vi "log analysis_gps.vi"() -> ()   [LabVIEW 2018] (continued)
15:20:57.4\tlog_raw\tgps_raw\t#DUALANTENNAHEADINGA,USB3,0,49.5,FINESTEERING,2107,282075.400,02000000,d426,15824;SOL_COMPUTED,L1_FLOAT,-1.000000000,190.728332520,52.272701263,0.0,209.958755493,180.000000000,\"631T\",21,7,7,7,04,00,20,02*2a740797\n\tsystem status\tnormal 2 28.100000 0 0\trobot status\t246.921443\t96.474986\t8.494500\t0.148213\t0.043685\t-28.674334\t0.301000\t0.002000\n\t\n15:20:57.9\tlog_raw\tgps_raw\t#DUALANTENNAHEADINGA,USB3,0,49.5,FINESTEERING,2107,282075.900,02000000,d426,15824;SOL_COMPUTED,L1_FLOAT,-1.000000000,190.868621826,51.534015656,0.0,206.683425903,180.000000000,\"631T\",14,7,7,7,04,00,20,03*060951e8\n\tsystem status\tnormal 2 28.100000 0 0\trobot status\t247.040258\t96.400033\t8.497000\t0.123898\t-0.129590\t-28.934715\t0.297000\t-0.013000\n\t\n15:20:58.4\tlog_raw\tgps_raw\t#DUALANTENNAHEADINGA,USB3,0,44.0,FINESTEERING,2107,282076.400,02000000,d426,15824;SOL_COMPUTED,NARROW_FLOAT,-1.000000000,164.765243530,-0.145935059,0.0,360.000000000,180.000000000,\"631T\",15,7,7,7,04,00,20,03*df327d6c\n\tsystem status\tnormal 2 28.100000 0 0\trobot status\t247.153173\t96.328172\t8.499300\t0.054880\t0.026721\t-29.154516\t0.311000\t0.002000\n\t\n15:20:58.9\tlog_raw\tgps_raw\t\tsystem status\tnormal 2 28.100000 0 0\trobot status\t247.265732\t96.255208\t8.500200\t0.112861\t0.355298\t-29.271130\t0.297000\t0.005000\n\t\n15:20:59.4\tlog_raw\tgps_raw\t\tsystem status\tnormal 2 28.100000 0 0\trobot status\t247.378509\t96.180954\t8.500400\t0.252561\t0.434005\t-29.420749\t0.301000\t0.008000\n\t\n15:20:59.9\tlog_raw\tgps_raw\t#DUALANTENNAHEADINGA,USB3,0,48.0,FINESTEERING,2107,282077.900,02000000,d426,15824;SOL_COMPUTED,NARROW_FLOAT,-1.000000000,163.219406128,-2.743896484,0.0,360.000000000,180.000000000,\"631T\",17,7,7,7,04,00,20,03*74221424\n\tsystem status\tnormal 2 28.100000 0 0\trobot status\t247.489808\t96.106361\t8.500700\t0.444252\t0.467575\t-29.545531\t0.301000\t0.005000\n\t\n15:21:00.4\tlog_raw\tgps_raw\t#DUALANTENNAHEADINGA,USB3,0,48.5,FINESTEERING,2107,282078.400,02000000,d426,15824;SOL_COMPUTED,NARROW_FLOAT,-1.000000000,164.756866455,-2.259979248,0.0,360.000000000,180.000000000,\"631T\",19,7,7,7,04,00,20,03*e2d4ab8a\n\tsystem status\tnormal 2 28.100000 0 0\trobot status\t247.603389\t96.030616\t8.501500\t0.397812\t0.362126\t-29.601914\t0.298000\t0.011000\n\t\n15:21:00.9\tlog_raw\tgps_raw\t#DUALANTENNAHEADINGA,USB3,0,48.5,FINESTEERING,2107,282078.900,02000000,d426,15824;SOL_COMPUTED,NARROW_FLOAT,-1.000000000,165.064834595,-2.246643066,0.0,360.000000000,180.000000000,\"631T\",18,7,7,7,04,00,20,03*e6e75529\n\tsystem status\tnormal 2 28.100000 0 0\trobot status\t247.723401\t95.952238\t8.502900\t0.211029\t0.110570\t-29.619450\t0.309000\t0.029000\n\t\n15:21:01.4\tlog_raw\tgps_raw\t#DUALANTENNAHEADINGA,USB3,0,47.5,FINESTEERING,2107,282079.400,02000000,d426,15824;SOL_COMPUTED,NARROW_FLOAT,-1.000000000,174.896926880,-30.356231689,0.0,360.000000000,180.000000000,\"631T\",18,7,7,7,04,00,20,03*d638673a\n\tsystem status\tnormal 2 28.100000 0 0\trobot status\t247.845096\t95.872152\t8.504300\t0.085021\t-0.119901\t-29.645623\t0.305000\t0.015000\n\t\n15:21:01.9\tlog_raw\tgps_raw\t#DUALANTENNAHEADINGA,USB3,0,47.5,FINESTEERING,2107,282079.900,02000000,d426,15824;SOL_COMPUTED,NARROW_FLOAT,-1.000000000,174.578781128,-31.075134277,0.0,360.000000000,180.000000000,\"631T\",17,7,7,7,04,00,20,03*d8acf742\n\tsystem status\tnormal 2 28.100000 0 0\trobot status\t247.963689\t95.793632\t8.505400\t-0.028469\t-0.053955\t-29.669528\t0.311000\t0.004000\n\t\n15:21:02.4\tlog_raw\tgps_raw\t\tsystem status\tnormal 2 28.100000 0 0\trobot status\t248.081422\t95.714785\t8.506300\t0.031084\t0.050569\t-29.647929\t0.294000\t0.017000\n\t\n15:21:02.9\tlog_raw\tgps_raw\t\tsystem status\tnormal 2 28.000000 0 0\trobot status\t248.195751\t95.637362\t8.506100\t0.171329\t0.096604\t-29.343964\t0.370000\t-0.086000\n\t\n15:21:03.4\tlog_raw\tgps_raw\t#DUALANTENNAHEADINGA,USB3,0,48.5,FINESTEERING,2107,282081.400,02000000,d426,15824;SOL_COMPUTED,NARROW_FLOAT,-1.000000000,186.002395630,72.538307190,0.0,360.000000000,180.000000000,\"631T\",18,7,7,7,04,00,20,02*94d40da5\n\tsystem status\tnormal 2 28.000000 0 0\trobot status\t248.312016\t95.561491\t8.506800\t0.012488\t0.198787\t-29.021105\t0.344000\t-0.051000\n\t\n15:21:03.9\tlog_raw\tgps_raw\t\tsystem status\tnormal 2 27.900000 0 0\trobot status\t248.431222\t95.484532\t8.507600\t-0.122842\t0.122402\t-28.483538\t0.262000\t0.063000\n\t\n15:21:04.4\tlog_raw\tgps_raw\t\tsystem status\tnormal 2 27.900000 0 0\trobot status\t248.548442\t95.409781\t8.509600\t-0.163692\t0.149809\t-27.878037\t0.300000\t0.006000\n\t\n15:21:04.9\tlog_raw\tgps_raw\t\tsystem status\tnormal 2 28.000000 0 0\trobot status\t248.667064\t95.335298\t8.510200\t-0.079262\t0.300498\t-27.192799\t0.222000\t0.147000\n\t\n15:21:05.4\tlog_raw\tgps_raw\t#INSPVAXA,USB3,0,48.0,FINESTEERING,2107,282083.450,02000000,471d,15824;INS_ALIGNMENT_COMPLETE,INS_RTKFIXED,37.37098848557,126.72364391635,8.5085,22.3000,-0.1545,0.2353,-0.0017,0.125081225,0.334802471,116.544491320,0.3966,0.2931,0.5085,0.1074,0.0919,0.0749,0.1481,0.1501,5.0097,0f000001,0*707b4fda\n\tsystem status\tnormal 2 28.000000 0 0\trobot status\t248.799900\t95.253167\t8.508500\t0.125081\t0.334802\t-26.544491\t0.294000\t0.032000\n\t\n15:21:05.9\tlog_raw\tgps_raw\t#INSPVAXA,USB3,0,48.0,FINESTEERING,2107,282083.950,02000000,471d,15824;INS_ALIGNMENT_COMPLETE,INS_RTKFIXED,37.37098781334,126.72364531945,8.5061,22.3000,-0.1397,0.2470,-0.0039,0.130744788,0.168821644,116.045699984,0.3966,0.2931,0.5085,0.1074,0.0919,0.0749,0.1481,0.1501,5.0097,0f000001,0*8c7cd4e3\n\tsystem status\tnormal 2 27.900000 0 0\trobot status\t248.924184\t95.178556\t8.506100\t0.130745\t0.168822\t-26.045700\t0.306000\t0.015000\n\t\n15:21:06.4\tlog_raw\tgps_raw\t#INSPVAXA,USB3,0,49.5,FINESTEERING,2107,282084.450,02000000,471d,15824;INS_ALIGNMENT_COMPLETE,INS_RTKFIXED,37.37098717814,126.72364671785,8.5044,22.3000,-0.1354,0.2435,-0.0138,-0.054756889,-0.022563669,115.524105800,0.3967,0.2930,0.5082,0.1073,0.0917,0.0749,0.1480,0.1501,5.0101,0f000001,0*e14fe85b\n\tsystem status\tnormal 2 28.000000 0 0\trobot status\t249.048052\t95.108055\t8.504400\t-0.054757\t-0.022564\t-25.524106\t0.397000\t-0.137000\n\t\n15:21:06.9\tlog_raw\tgps_raw\t#DUALANTENNAHEADINGA,USB3,0,49.5,FINESTEERING,2107,282084.900,02000000,d426,15824;SOL_COMPUTED,NARROW_FLOAT,-1.000000000,161.093994141,-39.642028809,0.0,360.000000000,180.000000000,\"631T\",18,7,7,7,04,00,20,02*551afc73\n\tsystem status\tnormal 2 28.000000 0 0\trobot status\t249.161436\t95.044023\t8.503800\t-0.170407\t-0.184756\t-25.155498\t0.339000\t-0.036000\n\t\n15:21:07.4\tlog_raw\tgps_raw\t\tsystem status\tnormal 2 28.000000 0 0\trobot status\t249.290152\t94.971247\t8.503100\t-0.112588\t-0.413886\t-24.896418\t0.198000\t0.158000\n\t\n15:21:07.9\tlog_raw\tgps_raw\t\tsystem status\tnormal 2 28.000000 0 0\trobot status\t249.416871\t94.899708\t8.501000\t-0.049468\t-0.480154\t-24.681244\t0.257000\t0.076000\n\t\n15:21:08.4\tlog_raw\tgps_raw\t\tsystem status\tnormal 2 28.000000 0 0\trobot status\t249.543697\t94.830890\t8.500800\t-0.123153\t-0.405635\t-24.666717\t0.251000\t0.079000\n\t\n15:21:08.9\tlog_raw\tgps_raw\t#INSPVAXA,USB3,0,45.5,FINESTEERING,2107,282086.950,02000000,471d,15824;INS_ALIGNMENT_COMPLETE,INS_RTKFIXED,37.37098400291,126.72365390857,8.5011,22.3000,-0.1413,0.2614,-0.0071,-0.222662760,-0.431667529,114.703885924,0.3961,0.2927,0.5077,0.1073,0.0916,0.0749,0.1479,0.1501,5.0112,0f000001,0*8c0cd5e8\n\tsystem status\tnormal 2 28.100000 0 0\trobot status\t249.684995\t94.755634\t8.501100\t-0.222663\t-0.431668\t-24.703886\t0.253000\t0.069000\n\t\n15:21:09.4\tlog_raw\tgps_raw\t\tsystem status\tnormal 2 28.100000 0 0\trobot status\t249.796178\t94.694217\t8.502700\t-0.161427\t-0.370643\t-24.781443\t0.302000\t-0.009000\n\t\n15:21:09.9\tlog_raw\tgps_raw\t#INSPVAXA,USB3,0,49.0,FINESTEERING,2107,282087.950,02000000,471d,15824;INS_ALIGNMENT_COMPLETE,INS_RTKFIXED,37.37098277282,126.72365670812,8.5043,22.3000,-0.1437,0.2560,-0.0135,-0.068385407,-0.323416769,114.901118705,0.3958,0.2926,0.5076,0.1072,0.0916,0.0749,0.1479,0.1502,5.0118,0f000001,0*c54dad40\n\tsystem status\tnormal 2 28.100000 0 0\trobot status\t249.932974\t94.619105\t8.504300\t-0.068385\t-0.323417\t-24.901119\t0.298000\t-0.013000\n\t\n15:21:10.4\tlog_raw\tgps_raw\t#INSPVAXA,USB3,0,45.0,FINESTEERING,2107,282088.450,02000000,471d,15824;INS_ALIGNMENT_COMPLETE,INS_RTKFIXED,37.37098213793,126.72365811830,8.5048,22.3000,-0.1404,0.2509,-0.0150,-0.140571199,-0.324537767,115.053900448,0.3958,0.2925,0.5075,0.1072,0.0917,0.0749,0.1479,0.1502,5.0126,0f000001,0*5d76f850\n\tsystem status\tnormal 2 28.100000 0 0\trobot status\t250.057886\t94.548639\t8.504800\t-0.140571\t-0.324538\t-25.053900\t0.300000\t-0.020000\n\t\n15:21:10.9\tlog_raw\tgps_raw\t\tsystem status\tnormal 2 28.100000 0 0\trobot status\t250.170070\t94.483065\t8.505900\t-0.049148\t-0.443713\t-25.152133\t0.309000\t-0.009000\n\t\n15:21:11.4\tlog_raw\tgps_raw\t\tsystem status\tnormal 2 28.100000 0 0\trobot status\t250.293447\t94.411259\t8.508800\t-0.003833\t-0.433412\t-25.288607\t0.296000\t-0.018000\n\t\n15:21:11.9\tlog_raw\tgps_raw\t#INSPVAXA,USB3,0,50.0,FINESTEERING,2107,282089.950,02000000,471d,15824;INS_ALIGNMENT_COMPLETE,INS_RTKFIXED,37.37098017514,126.72366234895,8.5129,22.3000,-0.1403,0.2638,-0.0115,0.068877400,-0.331025917,115.512688537,0.3958,0.2925,0.5074,0.1072,0.0917,0.0749,0.1479,0.1501,5.0134,0f000001,0*45d8cdd7\n\tsystem status\tnormal 2 28.100000 0 0\trobot status\t250.432630\t94.330788\t8.512900\t0.068877\t-0.331026\t-25.512689\t0.298000\t-0.016000\n\t\n15:21:12.4\tlog_raw\tgps_raw\t#INSPVAXA,USB3,0,47.0,FINESTEERING,2107,282090.450,02000000,471d,15824;INS_ALIGNMENT_COMPLETE,INS_RTKFIXED,37.37097950653,126.72366381280,8.5149,22.3000,-0.1497,0.2592,-0.0041,-0.040058431,-0.070783873,115.696569109,0.3958,0.2925,0.5072,0.1072,0.0918,0.0748,0.1480,0.1501,5.0142,0f000001,0*06fd62fb\n\tsystem status\tnormal 2 28.100000 0 0\trobot status\t250.562295\t94.256579\t8.514900\t-0.040058\t-0.070784\t-25.696569\t0.295000\t-0.015000\n\t\n15:21:12.9\tlog_raw\tgps_raw\t#DUALANTENNAHEADINGA,USB3,0,47.0,FINESTEERING,2107,282090.900,02000000,d426,15824;SOL_COMPUTED,NARROW_FLOAT,-1.000000000,171.721908569,34.681911469,0.0,360.000000000,180.000000000,\"631T\",20,7,7,7,04,00,20,03*da0d38e5\n\tsystem status\tnormal 2 28.100000 0 0\trobot status\t250.677266\t94.189308\t8.516000\t-0.049841\t0.271250\t-25.895908\t0.306000\t-0.016000\n\t\n15:21:13.4\tlog_raw\tgps_raw\t#INSPVAXA,USB3,0,47.0,FINESTEERING,2107,282091.450,02000000,471d,15824;INS_ALIGNMENT_COMPLETE,INS_RTKFIXED,37.37097820755,126.72366660545,8.5215,22.3000,-0.1497,0.2548,0.0005,-0.143132038,0.926627328,116.158649383,0.3959,0.2925,0.5072,0.1072,0.0918,0.0748,0.1480,0.1501,5.0152,0f000001,0*c99bd82f\n\tsystem status\tnormal 2 28.100000 0 0\trobot status\t250.809663\t94.112405\t8.521500\t-0.143132\t0.926627\t-26.158649\t0.299000\t-0.014000\n\t\n15:21:13.9\tlog_raw\tgps_raw\t#DUALANTENNAHEADINGA,USB3,0,47.0,FINESTEERING,2107,282091.900,02000000,d426,15824;SOL_COMPUTED,NARROW_FLOAT,-1.000000000,112.916130066,31.135679245,0.0,360.000000000,180.000000000,\"631T\",17,8,8,7,04,00,20,03*e78407cb\n\tsystem status\tnormal 2 28.100000 0 0\trobot status\t250.929101\t94.041496\t8.525700\t-0.018408\t0.996780\t-26.393163\t0.310000\t-0.006000\n\t\n15:21:14.4\tlog_raw\tgps_raw\t\tsystem status\tnormal 2 28.100000 0 0\trobot status\t251.054651\t93.967882\t8.529200\t-0.147378\t0.978647\t-26.703970\t0.302000\t-0.013000\n\t\n15:21:14.9\tlog_raw\tgps_raw\t#INSPVAXA,USB3,0,44.5,FINESTEERING,2107,282092.950,02000000,471d,15824;INS_ALIGNMENT_COMPLETE,INS_RTKFIXED,37.37097614467,126.72367094542,8.5349,22.3000,-0.1554,0.2816,0.0034,-0.093672408,0.920148848,117.196010792,0.3968,0.2926,0.5073,0.1073,0.0918,0.0749,0.1480,0.1500,5.0167,0f000001,0*78c5bf02\n\tsystem status\tnormal 2 28.100000 0 0\trobot status\t251.194091\t93.883445\t8.534900\t-0.093672\t0.920149\t-27.196011\t0.271000\t-0.056000\n\t\n15:21:15.4\tlog_raw\tgps_raw\t#INSPVAXA,USB3,0,49.0,FINESTEERING,2107,282093.450,02000000,471d,15824;INS_ALIGNMENT_COMPLETE,INS_RTKFIXED,37.37097543650,126.72367235664,8.5399,22.3000,-0.1638,0.2823,0.0033,-0.126887111,0.570236621,117.700862791,0.3975,0.2926,0.5072,0.1072,0.0917,0.0749,0.1480,0.1500,5.0184,0f000001,0*ead874db\n\tsystem status\tnormal 2 28.100000 0 0\trobot status\t251.319094\t93.804845\t8.539900\t-0.126887\t0.570237\t-27.700863\t0.283000\t-0.053000\n\t\n15:21:15.9\tlog_raw\tgps_raw\t#DUALANTENNAHEADINGA,USB3,0,49.0,FINESTEERING,2107,282093.900,02000000,d426,15824;SOL_COMPUTED,NARROW_FLOAT,-1.000000000,156.493606567,-47.281768799,0.0,360.000000000,180.000000000,\"631T\",19,7,7,7,04,00,20,03*77a80aac\n\tsystem status\tnormal 2 28.000000 0 0\trobot status\t251.432949\t93.733402\t8.545000\t-0.389248\t0.357754\t-28.088524\t0.278000\t-0.065000\n\t\n15:21:16.4\tlog_raw\tgps_raw\t\tsystem status\tnormal 2 28.000000 0 0\trobot status\t251.554090\t93.656544\t8.548800\t-0.417645\t0.623151\t-28.489175\t0.270000\t-0.059000\n\t\n15:21:16.9\tlog_raw\tgps_raw\t\tsystem status\tnormal 2 28.000000 0 0\trobot status\t251.675834\t93.577949\t8.555400\t-0.297721\t0.578023\t-28.861659\t0.303000\t-0.034000\n\t\n15:21:17.4\tlog_raw\tgps_raw\t\tsystem status\tnormal 2 28.100000 0 0\trobot status\t251.794007\t93.497874\t8.561500\t-0.057927\t0.756210\t-29.237305\t0.346000\t0.056000\n\t\n15:21:17.9\tlog_raw\tgps_raw\t\tsystem status\tnormal 2 28.100000 0 0\trobot status\t251.912469\t93.418342\t8.568300\t0.007452\t0.966597\t-29.571126\t0.263000\t-0.068000\n\t\n15:21:18.4\tlog_raw\tgps_raw\t\tsystem status\tnormal 2 28.100000 0 0\trobot status\t252.031352\t93.338903\t8.575100\t-0.062826\t1.099209\t-29.892121\t0.312000\t0.017000\n\t\n15:21:18.9\tlog_raw\tgps_raw\t#INSPVAXA,USB3,0,47.0,FINESTEERING,2107,282096.950,02000000,471d,15824;INS_ALIGNMENT_COMPLETE,INS_RTKFIXED,37.37097045983,126.72368185203,8.5832,22.3000,-0.1608,0.2476,0.0236,-0.099484529,1.317134321,120.192875691,0.3973,0.2927,0.5071,0.1071,0.0916,0.0748,0.1480,0.1498,5.0232,0f000001,0*5f8f6166\n\tsystem status\tnormal 2 28.100000 0 0\trobot status\t252.160181\t93.252486\t8.583200\t-0.099485\t1.317134\t-30.192876\t0.296000\t-0.007000\n\t\n15:21:19.4\tlog_raw\tgps_raw\t#INSPVAXA,USB3,0,49.5,FINESTEERING,2107,282097.450,02000000,471d,15824;INS_ALIGNMENT_COMPLETE,INS_RTKFIXED,37.37096974645,126.72368313135,8.5891,22.3000,-0.1610,0.2427,0.0162,-0.068092222,1.654408737,120.396603583,0.3975,0.2927,0.5071,0.1072,0.0917,0.0748,0.1480,0.1497,5.0248,0f000001,0*be15312d\n\tsystem status\tnormal 2 28.100000 0 0\trobot status\t252.273501\t93.173309\t8.589100\t-0.068092\t1.654409\t-30.396604\t0.298000\t0.002000\n\t\n15:21:19.9\tlog_raw\tgps_raw\t#INSPVAXA,USB3,0,49.5,FINESTEERING,2107,282097.950,02000000,471d,15824;INS_ALIGNMENT_COMPLETE,INS_RTKFIXED,37.37096903981,126.72368439114,8.5953,22.3000,-0.1607,0.2384,0.0184,-0.045725766,1.917999330,120.611516024,0.3975,0.2927,0.5071,0.1072,0.0917,0.0748,0.1480,0.1497,5.0248,0f000001,0*a51c9b7d\n\tsystem status\tnormal 2 28.100000 0 0\trobot status\t252.385091\t93.094879\t8.595300\t-0.045726\t1.917999\t-30.611516\t0.294000\t0.012000\n\t\n15:21:20.4\tlog_raw\tgps_raw\t\tsystem status\tnormal 2 28.100000 0 0\trobot status\t252.485041\t93.024301\t8.600700\t-0.033696\t2.207683\t-30.786207\t0.301000\t0.001000\n\t\n15:21:20.9\tlog_raw\tgps_raw\t#INSPVAXA,USB3,0,45.5,FINESTEERING,2107,282098.950,02000000,471d,15824;INS_ALIGNMENT_COMPLETE,INS_RTKFIXED,37.37096763192,126.72368689204,8.6086,22.3000,-0.1625,0.2437,0.0135,0.032441913,2.356888954,120.959811590,0.3979,0.2928,0.5071,0.1076,0.0919,0.0749,0.1479,0.1497,5.0261,0f000001,0*4f4ceb13\n\tsystem status\tnormal 2 28.100000 0 0\trobot status\t252.606616\t92.938618\t8.608600\t0.032442\t2.356889\t-30.959812\t0.298000\t0.007000\n\t\n15:21:21.4\tlog_raw\tgps_raw\t#INSPVAXA,USB3,0,49.5,FINESTEERING,2107,282099.450,02000000,471d,15824;INS_ALIGNMENT_COMPLETE,INS_RTKFIXED,37.37096691868,126.72368816492,8.6172,22.3000,-0.1639,0.2543,0.0151,0.021335732,2.482431048,120.995881908,0.3986,0.2930,0.5071,0.1077,0.0920,0.0749,0.1479,0.1497,5.0261,0f000001,0*203ab1e7\n\tsystem status\tnormal 2 28.100000 0 0\trobot status\t252.719366\t92.859456\t8.617200\t0.021336\t2.482431\t-30.995882\t0.298000\t0.011000\n\t\n15:21:21.9\tlog_raw\tgps_raw\t\tsystem status\tnormal 2 28.000000 0 0\trobot status\t252.825766\t92.786637\t8.625100\t-0.100390\t2.490390\t-30.971353\t0.296000\t0.007000\n\t\n15:21:22.4\tlog_raw\tgps_raw\t#INSPVAXA,USB3,0,48.5,FINESTEERING,2107,282100.450,02000000,471d,15824;INS_ALIGNMENT_COMPLETE,INS_RTKFIXED,37.37096543026,126.72369088215,8.6324,22.3000,-0.1596,0.2535,0.0180,-0.228914974,2.462239886,121.044086589,0.3992,0.2932,0.5070,0.1074,0.0920,0.0749,0.1478,0.1497,5.0245,0f000001,0*852ce3c8\n\tsystem status\tnormal 2 28.100000 0 0\trobot status\t252.960054\t92.694257\t8.632400\t-0.228915\t2.462240\t-31.044087\t0.302000\t0.006000\n\t\n15:21:22.9\tlog_raw\tgps_raw\t\tsystem status\tnormal 2 28.000000 0 0\trobot status\t253.065222\t92.621167\t8.638600\t-0.274642\t2.413490\t-30.976801\t0.306000\t0.011000\n\t\n15:21:23.4\tlog_raw\tgps_raw\t#INSPVAXA,USB3,0,48.5,FINESTEERING,2107,282101.450,02000000,471d,15824;INS_ALIGNMENT_COMPLETE,INS_RTKFIXED,37.37096396393,126.72369353310,8.6472,22.3000,-0.1601,0.2590,0.0331,-0.375730399,2.404420745,120.887856332,0.3993,0.2932,0.5070,0.1073,0.0921,0.0749,0.1478,0.1497,5.0225,0f000001,0*bfa232fa\n\tsystem status\tnormal 2 28.100000 0 0\trobot status\t253.194871\t92.531510\t8.647200\t-0.375730\t2.404421\t-30.887856\t0.302000\t0.009000\n\t\n15:21:23.9\tlog_raw\tgps_raw\t#INSPVAXA,USB3,0,48.5,FINESTEERING,2107,282101.950,02000000,471d,15824;INS_ALIGNMENT_COMPLETE,INS_RTKFIXED,37.37096322042,126.72369488771,8.6547,22.3000,-0.1481,0.2477,0.0237,-0.389461163,2.309809886,120.810766279,0.3993,0.2932,0.5070,0.1073,0.0921,0.0749,0.1478,0.1497,5.0225,0f000001,0*6153e896\n\tsystem status\tnormal 2 28.100000 0 0\trobot status\t253.314860\t92.448988\t8.654700\t-0.389461\t2.309810\t-30.810766\t0.357000\t-0.074000\n\t\n15:21:24.4\tlog_raw\tgps_raw\t#INSPVAXA,USB3,0,49.0,FINESTEERING,2107,282102.450,02000000,471d,15824;INS_ALIGNMENT_COMPLETE,INS_RTKFIXED,37.37096250169,126.72369619027,8.6639,22.3000,-0.1489,0.2563,0.0130,-0.492163713,2.419406589,120.611003212,0.3993,0.2933,0.5071,0.1074,0.0920,0.0750,0.1477,0.1497,5.0208,0f000001,0*e05fb414\n\tsystem status\tnormal 2 28.100000 0 0\trobot status\t253.430238\t92.369217\t8.663900\t-0.492164\t2.419407\t-30.611003\t0.264000\t0.072000\n\t\n15:21:24.9\tlog_raw\tgps_raw\t\tsystem status\tnormal 2 28.000000 0 0\trobot status\t253.533896\t92.296907\t8.672100\t-0.452442\t2.384637\t-30.249964\t0.449000\t-0.218000\n\t\n15:21:25.4\tlog_raw\tgps_raw\t#INSPVAXA,USB3,0,48.0,FINESTEERING,2107,282103.450,02000000,471d,15824;INS_ALIGNMENT_COMPLETE,INS_RTKFIXED,37.37096107043,126.72369881469,8.6799,22.3000,-0.1515,0.2464,0.0161,-0.632214670,2.279605302,119.849217483,0.3987,0.2933,0.5070,0.1074,0.0919,0.0750,0.1477,0.1496,5.0198,0f000001,0*6937ebdf\n\tsystem status\tnormal 2 28.000000 0 0\trobot status\t253.662705\t92.210362\t8.679900\t-0.632215\t2.279605\t-29.849217\t0.317000\t-0.014000\n\t\n15:21:25.9\tlog_raw\tgps_raw\t#INSPVAXA,USB3,0,48.0,FINESTEERING,2107,282103.950,02000000,471d,15824;INS_ALIGNMENT_COMPLETE,INS_RTKFIXED,37.37096036868,126.72370013653,8.6871,22.3000,-0.1575,0.2589,0.0105,-0.654965862,2.296906334,119.467685028,0.3987,0.2933,0.5070,0.1074,0.0919,0.0750,0.1477,0.1496,5.0198,0f000001,0*9d5844ee\n\tsystem status\tnormal 2 28.000000 0 0\trobot status\t253.779792\t92.132475\t8.687100\t-0.654966\t2.296906\t-29.467685\t0.368000\t-0.082000\n\t\n15:21:26.4\tlog_raw\tgps_raw\t\tsystem status\tnormal 2 28.000000 0 0\trobot status\t253.884722\t92.062093\t8.692300\t-0.660667\t2.168341\t-29.069913\t0.390000\t-0.123000\n\t\n15:21:26.9\tlog_raw\tgps_raw\t#INSPVAXA,USB3,0,48.5,FINESTEERING,2107,282104.950,02000000,471d,15824;INS_ALIGNMENT_COMPLETE,INS_RTKFIXED,37.37095896763,126.72370277535,8.6981,22.3000,-0.1486,0.2458,0.0269,-0.592987818,1.965751442,118.674591406,0.3980,0.2932,0.5070,0.1074,0.0918,0.0751,0.1476,0.1496,5.0196,0f000001,0*607cbc7a\n\tsystem status\tnormal 2 28.000000 0 0\trobot status\t254.013534\t91.976973\t8.698100\t-0.592988\t1.965751\t-28.674591\t0.372000\t-0.109000\n\t\n15:21:27.4\tlog_raw\tgps_raw\t#INSPVAXA,USB3,0,48.5,FINESTEERING,2107,282105.450,02000000,471d,15824;INS_ALIGNMENT_COMPLETE,INS_RTKFIXED,37.37095828575,126.72370408394,8.7035,22.3000,-0.1486,0.2405,0.0183,-0.703477485,1.966758993,118.307014299,0.3974,0.2931,0.5072,0.1076,0.0917,0.0751,0.1476,0.1496,5.0199,0f000001,0*e468851e\n\tsystem status\tnormal 2 27.900000 0 0\trobot status\t254.129447\t91.901291\t8.703500\t-0.703477\t1.966759\t-28.307014\t0.276000\t0.040000\n\t\n15:21:27.9\tlog_raw\tgps_raw\t#INSPVAXA,USB3,0,48.5,FINESTEERING,2107,282105.950,02000000,471d,15824;INS_ALIGNMENT_COMPLETE,INS_RTKFIXED,37.37095759805,126.72370541666,8.7095,22.3000,-0.1479,0.2589,0.0183,-0.776033189,1.928048544,118.044505224,0.3974,0.2931,0.5072,0.1076,0.0917,0.0751,0.1476,0.1496,5.0199,0f000001,0*d471bf4f\n\tsystem status\tnormal 2 28.000000 0 0\trobot status\t254.247497\t91.824963\t8.709500\t-0.776033\t1.928049\t-28.044505\t0.373000\t-0.111000\n\t\n15:21:28.4\tlog_raw\tgps_raw\t#INSPVAXA,USB3,0,46.5,FINESTEERING,2107,282106.450,02000000,471d,15824;INS_ALIGNMENT_COMPLETE,INS_RTKFIXED,37.37095690919,126.72370675668,8.7141,22.3000,-0.1377,0.2446,0.0099,-0.892542340,1.922749493,117.853154377,0.3968,0.2930,0.5072,0.1078,0.0917,0.0751,0.1476,0.1496,5.0204,0f000001,0*bc0c1e21\n\tsystem status\tnormal 2 28.000000 0 0\trobot status\t254.366194\t91.748507\t8.714100\t-0.892542\t1.922749\t-27.853154\t0.285000\t0.017000\n\t\n15:21:28.9\tlog_raw\tgps_raw\t#INSPVAXA,USB3,0,46.5,FINESTEERING,2107,282106.950,02000000,471d,15824;INS_ALIGNMENT_COMPLETE,INS_RTKFIXED,37.37095621502,126.72370811365,8.7176,22.3000,-0.1440,0.2520,0.0136,-0.957648564,1.997661807,117.680291492,0.3968,0.2930,0.5072,0.1078,0.0917,0.0751,0.1476,0.1496,5.0204,0f000001,0*5136ca20\n\tsystem status\tnormal 2 28.000000 0 0\trobot status\t254.486392\t91.671461\t8.717600\t-0.957649\t1.997662\t-27.680291\t0.350000\t-0.070000\n\t\n15:21:29.4\tlog_raw\tgps_raw\t#INSPVAXA,USB3,0,44.0,FINESTEERING,2107,282107.450,02000000,471d,15824;INS_ALIGNMENT_COMPLETE,INS_RTKFIXED,37.37095551506,126.72370946213,8.7227,22.3000,-0.1464,0.2502,0.0156,-0.936172746,1.990543984,117.627917664,0.3961,0.2929,0.5071,0.1075,0.0916,0.0751,0.1476,0.1496,5.0204,0f000001,0*d8872792\n\tsystem status\tnormal 2 28.100000 0 0\trobot status\t254.605838\t91.593773\t8.722700\t-0.936173\t1.990544\t-27.627918\t0.254000\t0.069000\n\t\n15:21:29.9\tlog_raw\tgps_raw\t#INSPVAXA,USB3,0,44.0,FINESTEERING,2107,282107.950,02000000,471d,15824;INS_ALIGNMENT_COMPLETE,INS_RTKFIXED,37.37095481415,126.72371079890,8.7282,22.3000,-0.1478,0.2544,0.0132,-0.866251632,1.815335912,117.612256060,0.3961,0.2929,0.5071,0.1075,0.0916,0.0751,0.1476,0.1496,5.0204,0f000001,0*57d0bda5\n\tsystem status\tnormal 2 28.100000 0 0\trobot status\t254.724247\t91.515979\t8.728200\t-0.866252\t1.815336\t-27.612256\t0.303000\t-0.008000\n\t\n15:21:30.4\tlog_raw\tgps_raw\t#INSPVAXA,USB3,0,47.5,FINESTEERING,2107,282108.450,02000000,471d,15824;INS_ALIGNMENT_COMPLETE,INS_RTKFIXED,37.37095411436,126.72371215377,8.7320,22.3000,-0.1500,0.2481,0.0140,-1.024789721,1.612981826,117.661458987,0.3956,0.2928,0.5070,0.1077,0.0917,0.0751,0.1475,0.1496,5.0202,0f000001,0*a0675bbc\n\tsystem status\tnormal 2 28.100000 0 0\trobot status\t254.832449\t91.445955\t8.731700\t-1.036836\t1.631412\t-27.629086\t0.309000\t-0.011000\n\t\n15:21:30.9\tlog_raw\tgps_raw\t#INSPVAXA,USB3,0,47.5,FINESTEERING,2107,282108.950,02000000,471d,15824;INS_ALIGNMENT_COMPLETE,INS_RTKFIXED,37.37095342524,126.72371347450,8.7365,22.3000,-0.1464,0.2522,0.0087,-1.211194385,1.652387786,117.710321786,0.3956,0.2928,0.5070,0.1077,0.0917,0.0751,0.1475,0.1496,5.0202,0f000001,0*fbbb71e9\n\tsystem status\tnormal 2 28.100000 0 0\trobot status\t254.961247\t91.361824\t8.736500\t-1.211194\t1.652388\t-27.710322\t0.300000\t-0.009000\n\t\n15:21:31.4\tlog_raw\tgps_raw\t#INSPVAXA,USB3,0,48.0,FINESTEERING,2107,282109.450,02000000,471d,15824;INS_ALIGNMENT_COMPLETE,INS_RTKFIXED,37.37095274133,126.72371479106,8.7424,22.3000,-0.1538,0.2512,0.0057,-1.183703798,1.673883858,117.732528128,0.3953,0.2928,0.5071,0.1077,0.0917,0.0751,0.1475,0.1496,5.0195,0f000001,0*a98a5245\n\tsystem status\tnormal 2 28.100000 0 0\trobot status\t255.077866\t91.285917\t8.742400\t-1.183704\t1.673884\t-27.732528\t0.299000\t-0.012000\n\t\n15:21:31.9\tlog_raw\tgps_raw\t#INSPVAXA,USB3,0,48.0,FINESTEERING,2107,282109.950,02000000,471d,15824;INS_ALIGNMENT_COMPLETE,INS_RTKFIXED,37.37095203304,126.72371616104,8.7487,22.3000,-0.1514,0.2528,0.0147,-1.036882261,1.559922655,117.777953155,0.3953,0.2928,0.5071,0.1077,0.0917,0.0751,0.1475,0.1496,5.0195,0f000001,0*d50cd7f7\n\tsystem status\tnormal 2 28.100000 0 0\trobot status\t255.199216\t91.207304\t8.748700\t-1.036882\t1.559923\t-27.777953\t0.298000\t-0.010000\n\t\n15:21:32.4\tlog_raw\tgps_raw\t#INSPVAXA,USB3,0,48.5,FINESTEERING,2107,282110.450,02000000,471d,15824;INS_ALIGNMENT_COMPLETE,INS_RTKFIXED,37.37095133527,126.72371748883,8.7530,22.3000,-0.1494,0.2469,0.0119,-1.026348823,1.537323059,117.877652049,0.3951,0.2928,0.5070,0.1077,0.0917,0.0751,0.1475,0.1496,5.0182,0f000001,0*ecbd9d89\n\tsystem status\tnormal 2 28.100000 0 0\trobot status\t255.316830\t91.129859\t8.753000\t-1.026349\t1.537323\t-27.877652\t0.294000\t-0.012000\n\t\n15:21:32.9\tlog_raw\tgps_raw\t#INSPVAXA,USB3,0,48.5,FINESTEERING,2107,282110.950,02000000,471d,15824;INS_ALIGNMENT_COMPLETE,INS_RTKFIXED,37.37095063141,126.72371883736,8.7567,22.3000,-0.1443,0.2312,0.0129,-1.128303497,1.542678809,118.026662583,0.3951,0.2928,0.5070,0.1077,0.0917,0.0751,0.1475,0.1496,5.0182,0f000001,0*daaca067\n\tsystem status\tnormal 2 28.100000 0 0\trobot status\t255.436280\t91.051737\t8.756700\t-1.128303\t1.542679\t-28.026663\t0.300000\t-0.015000\n\t\n15:21:33.4\tlog_raw\tgps_raw\t#INSPVAXA,USB3,0,46.0,FINESTEERING,2107,282111.450,02000000,471d,15824;INS_ALIGNMENT_COMPLETE,INS_RTKFIXED,37.37094994978,126.72372015306,8.7620,22.3000,-0.1561,0.2454,0.0089,-1.155550094,1.466986679,118.115120191,0.3996,0.2955,0.5135,0.1085,0.0924,0.0757,0.1476,0.1497,5.0168,0f000001,0*9d755c1d\n\tsystem status\tnormal 2 28.100000 0 0\trobot status\t255.552823\t90.976083\t8.762000\t-1.155550\t1.466987\t-28.115120\t0.294000\t-0.012000\n\t\n15:21:33.9\tlog_raw\tgps_raw\t#INSPVAXA,USB3,0,46.0,FINESTEERING,2107,282111.950,02000000,471d,15824;INS_ALIGNMENT_COMPLETE,INS_RTKFIXED,37.37094924686,126.72372148621,8.7667,22.3000,-0.1592,0.2411,0.0080,-1.003376747,1.533507787,118.272208873,0.3996,0.2955,0.5135,0.1085,0.0924,0.0757,0.1476,0.1497,5.0168,0f000001,0*68376ab3\n\tsystem status\tnormal 2 28.100000 0 0\trobot status\t255.670911\t90.898066\t8.766700\t-1.003377\t1.533508\t-28.272209\t0.297000\t-0.009000\n\t\n15:21:34.4\tlog_raw\tgps_raw\t\tsystem status\tnormal 2 28.100000 0 0\trobot status\t255.789718\t90.818730\t8.771500\t-0.873360\t1.552443\t-28.483035\t0.296000\t-0.012000\n\t\n15:21:34.9\tlog_raw\tgps_raw\t\tsystem status\tnormal 2 28.100000 0 0\trobot status\t255.906056\t90.740294\t8.777100\t-0.808408\t1.619075\t-28.703689\t0.300000\t-0.012000\n\t\n15:21:35.4\tlog_raw\tgps_raw\t#INSPVAXA,USB3,0,47.5,FINESTEERING,2107,282113.450,02000000,471d,15824;INS_ALIGNMENT_COMPLETE,INS_RTKFIXED,37.37094709383,126.72372548494,8.7822,22.3000,-0.1691,0.2475,0.0112,-0.824972405,1.586356961,118.983770593,0.4030,0.2950,0.5178,0.1084,0.0922,0.0757,0.1475,0.1497,5.0138,0f000001,0*59439988\n\tsystem status\tnormal 2 28.100000 0 0\trobot status\t256.025112\t90.659102\t8.782200\t-0.824972\t1.586357\t-28.983771\t0.301000\t-0.011000\n\t\n15:21:35.9\tlog_raw\tgps_raw\t\tsystem status\tnormal 2 28.100000 0 0\trobot status\t256.144022\t90.575634\t8.786900\t-0.702476\t1.457846\t-29.249022\t0.300000\t-0.016000\n\t\n15:21:36.4\tlog_raw\tgps_raw\t\tsystem status\tnormal 2 28.100000 0 0\trobot status\t256.264460\t90.491355\t8.790800\t-0.676967\t1.349210\t-29.497419\t0.298000\t-0.010000\n\t\n15:21:36.9\tlog_raw\tgps_raw\t#INSPVAXA,USB3,0,51.5,FINESTEERING,2107,282114.950,02000000,471d,15824;INS_ALIGNMENT_COMPLETE,INS_RTKFIXED,37.37094483188,126.72372951627,8.7947,22.3000,-0.1730,0.2314,0.0140,-0.653922567,1.323648308,119.738020967,0.4016,0.2936,0.5159,0.1080,0.0922,0.0755,0.1474,0.1496,5.0125,0f000001,0*093f9180\n\tsystem status\tnormal 2 28.100000 0 0\trobot status\t256.382201\t90.408050\t8.794700\t-0.653923\t1.323648\t-29.738021\t0.296000\t-0.003000\n\t\n15:21:37.4\tlog_raw\tgps_raw\t#INSPVAXA,USB3,0,50.5,FINESTEERING,2107,282115.450,02000000,471d,15824;INS_ALIGNMENT_COMPLETE,INS_RTKFIXED,37.37094409692,126.72373081199,8.8000,22.3000,-0.1872,0.2511,0.0165,-0.607846314,1.413014132,119.977031024,0.3998,0.2929,0.5140,0.1075,0.0920,0.0753,0.1474,0.1495,5.0103,0f000001,0*d87b3f60\n\tsystem status\tnormal 2 28.100000 0 0\trobot status\t256.496974\t90.326477\t8.800000\t-0.607846\t1.413014\t-29.977031\t0.302000\t-0.012000\n\t\n15:21:37.9\tlog_raw\tgps_raw\t#INSPVAXA,USB3,0,50.5,FINESTEERING,2107,282115.950,02000000,471d,15824;INS_ALIGNMENT_COMPLETE,INS_RTKFIXED,37.37094333872,126.72373213439,8.8049,22.3000,-0.1750,0.2376,0.0100,-0.458555016,1.505006128,120.195242243,0.3998,0.2929,0.5140,0.1075,0.0920,0.0753,0.1474,0.1495,5.0103,0f000001,0*9085454d\n\tsystem status\tnormal 2 28.100000 0 0\trobot status\t256.614110\t90.242325\t8.804900\t-0.458555\t1.505006\t-30.195242\t0.296000\t-0.001000\n\t\n15:21:38.4\tlog_raw\tgps_raw\t#INSPVAXA,USB3,0,47.5,FINESTEERING,2107,282116.450,02000000,471d,15824;INS_ALIGNMENT_COMPLETE,INS_RTKFIXED,37.37094260633,126.72373343529,8.8096,22.3000,-0.1820,0.2326,0.0074,-0.394320906,1.730091512,120.395772522,0.3983,0.2926,0.5122,0.1073,0.0921,0.0752,0.1473,0.1495,5.0085,0f000001,0*0af836cc\n\tsystem status\tnormal 2 28.100000 0 0\trobot status\t256.729341\t90.161037\t8.809600\t-0.394321\t1.730092\t-30.395773\t0.298000\t0.000000\n\t\n15:21:38.9\tlog_raw\tgps_raw\t#INSPVAXA,USB3,0,47.5,FINESTEERING,2107,282116.950,02000000,471d,15824;INS_ALIGNMENT_COMPLETE,INS_RTKFIXED,37.37094186601,126.72373474956,8.8141,22.3000,-0.1805,0.2419,0.0176,-0.396545512,1.701319201,120.653391507,0.3983,0.2926,0.5122,0.1073,0.0921,0.0752,0.1473,0.1495,5.0085,0f000001,0*1c5a80aa\n\tsystem status\tnormal 2 28.100000 0 0\trobot status\t256.845757\t90.078870\t8.814100\t-0.396546\t1.701319\t-30.653392\t0.298000\t-0.001000\n\t\n15:21:39.4\tlog_raw\tgps_raw\t#INSPVAXA,USB3,0,50.0,FINESTEERING,2107,282117.450,02000000,471d,15824;INS_ALIGNMENT_COMPLETE,INS_RTKFIXED,37.37094111146,126.72373605556,8.8178,22.3000,-0.1868,0.2460,0.0165,-0.381592646,1.647549493,120.846709462,0.3974,0.2926,0.5106,0.1073,0.0921,0.0751,0.1472,0.1494,5.0066,0f000001,0*ba01e3a8\n\tsystem status\tnormal 2 28.100000 0 0\trobot status\t256.961440\t89.995123\t8.817800\t-0.381593\t1.647549\t-30.846709\t0.300000\t-0.003000\n\t\n15:21:39.9\tlog_raw\tgps_raw\t#INSPVAXA,USB3,0,50.0,FINESTEERING,2107,282117.950,02000000,471d,15824;INS_ALIGNMENT_COMPLETE,INS_RTKFIXED,37.37094033819,126.72373738098,8.8215,22.3000,-0.1807,0.2431,0.0157,-0.357927005,1.593594515,120.982465037,0.3974,0.2926,0.5106,0.1073,0.0921,0.0751,0.1472,0.1494,5.0066,0f000001,0*473a97aa\n\tsystem status\tnormal 2 28.100000 0 0\trobot status\t257.078844\t89.909298\t8.821500\t-0.357927\t1.593595\t-30.982465\t0.299000\t0.000000\n\t\n15:21:40.4\tlog_raw\tgps_raw\t#INSPVAXA,USB3,0,47.0,FINESTEERING,2107,282118.450,02000000,471d,15824;INS_ALIGNMENT_COMPLETE,INS_RTKFIXED,37.37093956964,126.72373870165,8.8242,22.3000,-0.1812,0.2503,0.0145,-0.278070640,1.434405224,121.098239314,0.3976,0.2926,0.5095,0.1073,0.0920,0.0750,0.1472,0.1494,5.0051,0f000001,0*4b2331c4\n\tsystem status\tnormal 2 28.100000 0 0\trobot status\t257.195827\t89.823997\t8.824200\t-0.278071\t1.434405\t-31.098239\t0.303000\t0.004000\n\t\n15:21:40.9\tlog_raw\tgps_raw\t#INSPVAXA,USB3,0,47.0,FINESTEERING,2107,282118.950,02000000,471d,15824;INS_ALIGNMENT_COMPLETE,INS_RTKFIXED,37.37093879764,126.72374003076,8.8271,22.3000,-0.1824,0.2531,0.0181,-0.239679007,1.415709773,121.121487507,0.3976,0.2926,0.5095,0.1073,0.0920,0.0750,0.1472,0.1494,5.0051,0f000001,0*31152a6b\n\tsystem status\tnormal 2 28.100000 0 0\trobot status\t257.313557\t89.738314\t8.827100\t-0.239679\t1.415710\t-31.121488\t0.302000\t0.007000\n\t\n15:21:41.4\tlog_raw\tgps_raw\t\tsystem status\tnormal 2 28.100000 0 0\trobot status\t257.429454\t89.653528\t8.831000\t-0.210575\t1.455050\t-31.151179\t0.294000\t0.006000\n\t\n15:21:41.9\tlog_raw\tgps_raw\t#INSPVAXA,USB3,0,51.0,FINESTEERING,2107,282119.950,02000000,471d,15824;INS_ALIGNMENT_COMPLETE,INS_RTKFIXED,37.37093727154,126.72374264951,8.8356,22.3000,-0.1820,0.2425,0.0126,-0.263751885,1.526286422,121.184806545,0.3974,0.2926,0.5086,0.1074,0.0920,0.0750,0.1471,0.1494,5.0040,0f000001,0*c7b594c4\n\tsystem status\tnormal 2 28.100000 0 0\trobot status\t257.545522\t89.568933\t8.835600\t-0.263752\t1.526286\t-31.184807\t0.300000\t0.003000\n\t\n15:21:42.4\tlog_raw\tgps_raw\t\tsystem status\tnormal 2 28.100000 0 0\trobot status\t257.663467\t89.482263\t8.840000\t-0.150267\t1.442051\t-31.195253\t0.297000\t0.002000\n\t\n15:21:42.9\tlog_raw\tgps_raw\t\tsystem status\tnormal 2 28.100000 0 0\trobot status\t257.780189\t89.397460\t8.843700\t-0.211609\t1.524071\t-31.245965\t0.293000\t0.001000\n\t\n15:21:43.4\tlog_raw\tgps_raw\t\tsystem status\tnormal 2 28.100000 0 0\trobot status\t257.897045\t89.313035\t8.847200\t-0.292123\t1.512764\t-31.266268\t0.294000\t0.006000\n\t\n15:21:43.9\tlog_raw\tgps_raw\t#INSPVAXA,USB3,0,49.5,FINESTEERING,2107,282121.950,02000000,471d,15824;INS_ALIGNMENT_COMPLETE,INS_RTKFIXED,37.37093422508,126.72374790381,8.8513,22.3000,-0.1769,0.2415,0.0095,-0.361327537,1.582717888,121.199299020,0.3976,0.2927,0.5074,0.1074,0.0918,0.0750,0.1470,0.1494,5.0032,0f000001,0*bd59e65f\n\tsystem status\tnormal 2 28.100000 0 0\trobot status\t258.010939\t89.230808\t8.851300\t-0.361328\t1.582718\t-31.199299\t0.296000\t0.007000\n\t\n15:21:44.4\tlog_raw\tgps_raw\t\tsystem status\tnormal 2 28.100000 0 0\trobot status\t258.127203\t89.146683\t8.855700\t-0.347219\t1.693226\t-31.178397\t0.279000\t0.041000\n\t\n15:21:44.9\tlog_raw\tgps_raw\t#INSPVAXA,USB3,0,51.5,FINESTEERING,2107,282122.950,02000000,471d,15824;INS_ALIGNMENT_COMPLETE,INS_RTKFIXED,37.37093271089,126.72375052599,8.8596,22.3000,-0.1652,0.2321,0.0060,-0.281890113,1.847721307,121.184840630,0.3974,0.2927,0.5070,0.1074,0.0918,0.0750,0.1469,0.1494,5.0040,0f000001,0*3de7c804\n\tsystem status\tnormal 2 28.100000 0 0\trobot status\t258.243207\t89.062749\t8.859600\t-0.281890\t1.847721\t-31.184841\t0.291000\t0.006000\n\t\n15:21:45.4\tlog_raw\tgps_raw\t\tsystem status\tnormal 2 28.100000 0 0\trobot status\t258.360298\t88.980183\t8.864400\t-0.326618\t1.910174\t-31.140281\t0.344000\t-0.067000\n\t\n15:21:45.9\tlog_raw\tgps_raw\t\tsystem status\tnormal 2 28.000000 0 0\trobot status\t258.477914\t88.899959\t8.869800\t-0.566893\t1.971210\t-31.050375\t0.291000\t0.013000\n\t\n15:21:46.4\tlog_raw\tgps_raw\t\tsystem status\tnormal 2 28.000000 0 0\trobot status\t258.594927\t88.819508\t8.876000\t-0.705882\t2.053406\t-30.885197\t0.301000\t0.019000\n\t\n15:21:46.9\tlog_raw\tgps_raw\t\tsystem status\tnormal 2 28.000000 0 0\trobot status\t258.711010\t88.739806\t8.881400\t-0.716451\t2.150721\t-30.754732\t0.296000\t0.028000\n\t\n15:21:47.4\tlog_raw\tgps_raw\t\tsystem status\tnormal 2 28.100000 0 0\trobot status\t258.828042\t88.660108\t8.886100\t-0.665736\t2.204894\t-30.635162\t0.294000\t0.020000\n\t\n15:21:47.9\tlog_raw\tgps_raw\t\tsystem status\tnormal 2 28.000000 0 0\trobot status\t258.944428\t88.582420\t8.892000\t-0.755659\t2.373283\t-30.507484\t0.288000\t0.025000\n\t\n15:21:48.4\tlog_raw\tgps_raw\t\tsystem status\tnormal 2 28.000000 0 0\trobot status\t259.060311\t88.502698\t8.896400\t-0.725355\t2.248232\t-30.402934\t0.267000\t0.041000\n\t\n15:21:48.9\tlog_raw\tgps_raw\t\tsystem status\tnormal 2 28.000000 0 0\trobot status\t259.178415\t88.422560\t8.901400\t-0.805729\t2.094399\t-30.405427\t0.278000\t0.020000\n\t\n15:21:49.4\tlog_raw\tgps_raw\t\tsystem status\tnormal 2 28.100000 0 0\trobot status\t259.297409\t88.341572\t8.908100\t-0.871560\t2.116869\t-30.395366\t0.286000\t-0.002000\n\t\n15:21:49.9\tlog_raw\tgps_raw\t\tsystem status\tnormal 2 28.100000 0 0\trobot status\t259.417089\t88.259389\t8.913700\t-0.840026\t1.936456\t-30.417131\t0.300000\t-0.010000\n\t\n15:21:50.4\tlog_raw\tgps_raw\t\tsystem status\tnormal 2 28.100000 0 0\trobot status\t259.531609\t88.179415\t8.921500\t-0.616551\t1.740916\t-30.413226\t0.300000\t-0.007000\n\t\n15:21:50.9\tlog_raw\tgps_raw\t\tsystem status\tnormal 2 28.100000 0 0\trobot status\t259.646947\t88.100247\t8.929200\t-0.589958\t1.982721\t-30.414505\t0.298000\t-0.007000\n\t\n15:21:51.4\tlog_raw\tgps_raw\t\tsystem status\tnormal 2 28.100000 0 0\trobot status\t259.760550\t88.020418\t8.935400\t-0.618112\t1.918967\t-30.411558\t0.302000\t-0.007000\n\t\n15:21:51.9\tlog_raw\tgps_raw\t\tsystem status\tnormal 2 28.000000 0 0\trobot status\t259.873198\t87.942660\t8.942100\t-0.787968\t2.032366\t-30.407234\t0.305000\t-0.004000\n\t\n15:21:52.4\tlog_raw\tgps_raw\t\tsystem status\tnormal 2 28.100000 0 0\trobot status\t259.985688\t87.862064\t8.948100\t-0.661636\t2.302182\t-30.434015\t0.299000\t-0.012000\n\t\n15:21:52.9\tlog_raw\tgps_raw\t\tsystem status\tnormal 2 28.100000 0 0\trobot status\t260.101413\t87.779957\t8.955000\t-0.617017\t2.234613\t-30.506198\t0.297000\t-0.012000\n\t\n15:21:53.4\tlog_raw\tgps_raw\t\tsystem status\tnormal 2 28.100000 0 0\trobot status\t260.218060\t87.697438\t8.963500\t-0.592380\t2.173030\t-30.665294\t0.307000\t-0.010000\n\t\n15:21:53.9\tlog_raw\tgps_raw\t\tsystem status\tnormal 2 28.100000 0 0\trobot status\t260.333259\t87.615710\t8.972100\t-0.604449\t2.150564\t-30.874121\t0.303000\t-0.010000\n\t\n15:21:54.4\tlog_raw\tgps_raw\t\tsystem status\tnormal 2 28.100000 0 0\trobot status\t260.449233\t87.531925\t8.979400\t-0.722415\t2.067451\t-31.097111\t0.298000\t-0.009000\n\t\n15:21:54.9\tlog_raw\tgps_raw\t\tsystem status\tnormal 2 28.100000 0 0\trobot status\t260.565612\t87.446785\t8.986300\t-0.763202\t2.269904\t-31.311944\t0.302000\t-0.012000\n\t\n15:21:55.4\tlog_raw\tgps_raw\t\tsystem status\tnormal 2 28.100000 0 0\trobot status\t260.680104\t87.362737\t8.994100\t-0.817055\t2.239245\t-31.507276\t0.294000\t-0.007000\n\t\n15:21:55.9\tlog_raw\tgps_raw\t\tsystem status\tnormal 2 28.100000 0 0\trobot status\t260.796658\t87.276263\t9.001600\t-0.792363\t2.059888\t-31.728451\t0.295000\t-0.006000\n\t\n15:21:56.4\tlog_raw\tgps_raw\t\tsystem status\tnormal 2 28.100000 0 0\trobot status\t260.914432\t87.187958\t9.009000\t-0.759293\t1.874172\t-31.924971\t0.293000\t0.002000\n\t\n15:21:56.9\tlog_raw\tgps_raw\t\tsystem status\tnormal 2 28.100000 0 0\trobot status\t261.029756\t87.100716\t9.017700\t-0.708694\t1.759464\t-32.163681\t0.299000\t-0.006000\n\t\n15:21:57.4\tlog_raw\tgps_raw\t\tsystem status\tnormal 2 28.100000 0 0\trobot status\t261.145843\t87.012287\t9.024600\t-0.771549\t1.613493\t-32.379821\t0.300000\t-0.003000\n\t\n15:21:57.9\tlog_raw\tgps_raw\t\tsystem status\tnormal 2 28.100000 0 0\trobot status\t261.261864\t86.924514\t9.030500\t-0.914921\t1.506825\t-32.551536\t0.301000\t0.000000\n\t\n15:21:58.4\tlog_raw\tgps_raw\t\tsystem status\tnormal 2 28.100000 0 0\trobot status\t261.376012\t86.837405\t9.035100\t-1.015951\t1.611516\t-32.716195\t0.304000\t-0.003000\n\t\n15:21:58.9\tlog_raw\tgps_raw\t\tsystem status\tnormal 2 28.100000 0 0\trobot status\t261.487677\t86.750445\t9.040100\t-0.945228\t1.574798\t-32.811251\t0.298000\t0.000000\n\t\n15:21:59.4\tlog_raw\tgps_raw\t\tsystem status\tnormal 2 28.100000 0 0\trobot status\t261.599992\t86.663449\t9.046200\t-0.911916\t1.440569\t-32.861815\t0.305000\t0.003000\n\t\n15:21:59.9\tlog_raw\tgps_raw\t\tsystem status\tnormal 2 28.100000 0 0\trobot status\t261.713949\t86.575535\t9.052100\t-0.901610\t1.511680\t-32.859544\t0.293000\t0.003000\n\t\n15:22:00.4\tlog_raw\tgps_raw\t\tsystem status\tnormal 2 28.100000 0 0\trobot status\t261.829812\t86.486788\t9.056900\t
